vi "updatedFile RawTestSelect.vi"(6 "Column Number":u32=21, 8 "Selected Index":dbl[](array[numeric]), 11 "Path":path=path "C:/Users/Flash/Desktop/Data/Detector test data/A-3355-3-A_Diode_Full_300_20171020092832.csv") -> ()   [LabVIEW 2012]
uses:
  <vilib>/Utility/file.llb/Read From Spreadsheet File (string).vi
  <vilib>/Utility/file.llb/Write To Spreadsheet File (string).vi
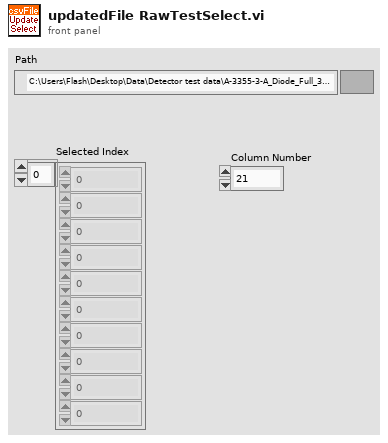
[diagram p1: front panel]
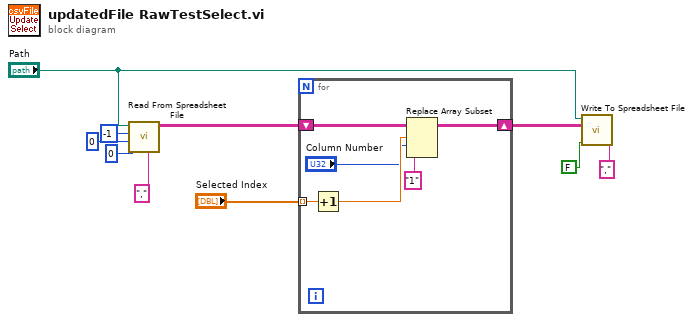
[diagram p0: block diagram]
diagram:
  n1 = call-poly <vilib>:"Read From Spreadsheet File.vi"("delimiter (\\t)"="," ("delimiter (\\t)"), "max characters/row  (no limit:0)"=0, "start of read offset (chars.:0)"=0, "number of rows (all:-1)"=-1, "file path (dialog if empty)"="Path") -> ("all rows"=w9:string[][])  [unwired: 2 in, 4 out]
  n2 = for {
    tunnel: "Selected Index" -> [w13] mode=indexing
    shift-right: [w14] -> w1
    shift-left: w9 -> [w16]
    n3 = Increment(x=w13) -> (x+1=w12:dbl)
    n4 = Replace Array Subset(array=w16, new element="1" ("new element/subarray"), index (row)=w12, index (col)="Column Number") -> (w14:string[][])
  }
  n5 = call-poly <vilib>:"Write To Spreadsheet File.vi"("delimiter (\\t)"="," ("delimiter (\\t)"), "append to file? (new file:F)"=FALSE, "2D data"=w1, "file path (dialog if empty)"="Path") -> ()  [unwired: 4 in, 1 out]
